vi "Write RFFE_w_Waveform.vi"(7 "Pins":string[](array[string])=["CLK", "SDA"], 8 "error in (no error)":errorcluster, 9 "Reg_Address_Data":T2={"Address"=81, "Data"=0} {"Address" format="%.0x"}, 10 "USID":T3 max=15, 11 "Semiconductor Module Context":T4) -> (0 "error out":errorcluster)   [LabVIEW 2013]
uses:
  <vilib>/NI_TestStand_SemiconductorModule/NI_TestStand_Semiconductor_Module.lvlibp/PinMap/General/SemiconductorModuleContext.ctl
  Controls/USID.ctl
  Controls/Reg_Address_Data.ctl
  MIPI_RFFE/Ctrls/RegReadWrite.ctl
  MIPI_RFFE/Ctrls/Configuration.ctl
  MIPI_RFFE/Ctrls/ClockDataChannels.ctl
  MIPI_RFFE/Ctrls/ExtendedRegReadWrite.ctl
  <instrlib>/niHSDIO/niHSDIO.llb/niHSDIO_ctl Generation Mode Values (Ring).ctl
  <vilib>/NI_TestStand_SemiconductorModule/NI_TestStand_Semiconductor_Module.lvlibp/PinMap/HSDIO/PinsToNIHSDIOSessions.vi
  <instrlib>/niHSDIO/niHSDIO.llb/niHSDIO Write Named Waveform (WDT).vi
  <vilib>/NI_TestStand_SemiconductorModule/NI_TestStand_Semiconductor_Module.lvlibp
panel:
  out "Converted Data":T1 {"Register" max=31 format="%.0x"; "Slave Address" max=15 format="%.0x"}
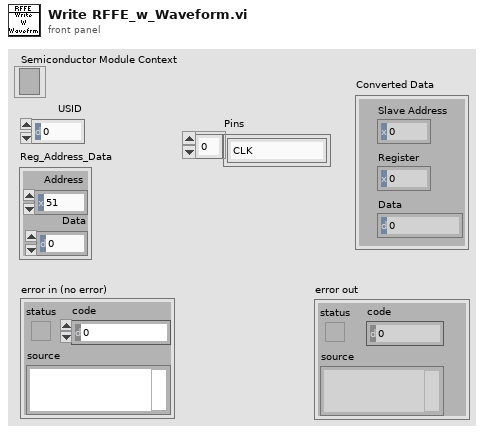
[diagram p1: front panel]
types:
  T1 = cluster{"Slave Address":u8, "Register":u8, "Data":u8}
  T2 = typedef "Reg_Address_Data.ctl" = cluster{"Address":u8, "Data":u8}
  T3 = typedef "USID.ctl" = u8
  T4 = typedef "NI_TestStand_Semiconductor_Module.lvlibp/SemiconductorModuleContext.ctl" = refnum<k7>
  T5 = typedef "Configuration.ctl" = cluster{"Samples to Allocate":i32, "Oversample Factor":u8, "Clock Channel":T6, "Data Channel":T6}
  T6 = typedef "ClockDataChannels.ctl" = enum16{"0", "1"}
  T7 = typedef "RegReadWrite.ctl" = cluster{"Slave Address":u8, "Register":u8, "Data":u8, "SetID_Pin_State":enum16{"0", "1", "Z"}}
  T8 = typedef "RFFE_Data.ctl" = cluster{"Clock Channel":T6, "Data Channel":T6, "Oversample Factor":u8, "Zero Array":u8[], "One Array":u8[], "Z Array ":u8[], "H Array":u8[], "L Array":u8[], "X Array":u8[], "Toggle (high to low)":u8[]}
  T9 = typedef "ExtendedRegReadWrite.ctl" = cluster{"Slave Address":u8, "Register":u8, "Data":u8[]}
  T10 = typedef "niHSDIO_ctl Generation Mode Values (Ring).ctl" = i32
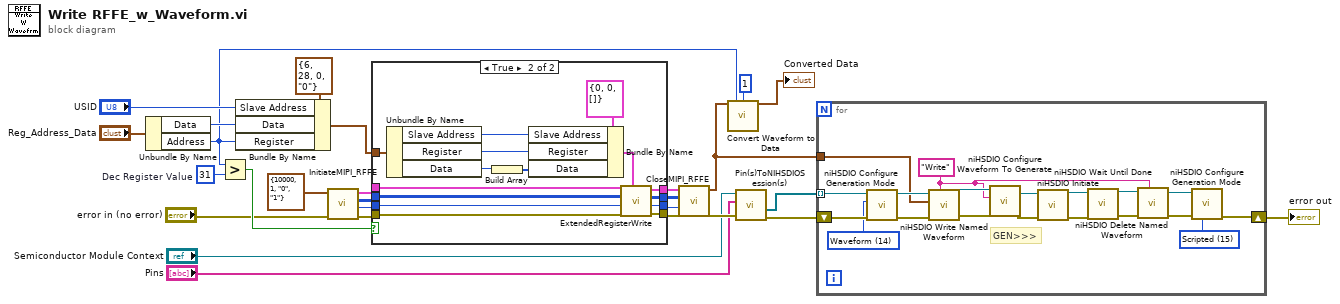
[diagram p0: block diagram]
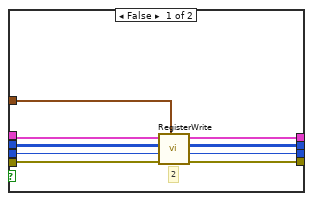
[diagram p2: hidden frame]
diagram:
  w23 = u8 31  # Dec Register Value
  n1 = Unbundle By Name("Reg_Address_Data") -> ("Data"=w5:u8, "Address"=w3:u8)
  n2 = Greater?(x=w3, y=w23) -> (0:w17:bool)
  n3 = Bundle By Name(cluster=T7 {"Slave Address"=6, "Register"=28, "Data"=0, "SetID_Pin_State"=enum."0"} ("Data"), "Slave Address"="USID", "Data"=w5, "Register"=w3) -> (w8:T7)
  n4 = call "InitiateMIPI_RFFE.vi"("error in (no error)"="error in (no error)", "Configuratation In"=T5 {"Samples to Allocate"=10000, "Oversample Factor"=1, "Clock Channel"=enum."0", "Data Channel"=enum."1"} ("Configuratation")) -> ("error out"=w16:errorcluster, "Number of Samples Out"=w15:i32, "Data Array"=w14:u8[][], "RFFE_Data"=w13:T8)  [unwired: 6 in]
  n5 = case shown="True" w17 {
    tunnel: [w31 w41] -> w22
    tunnel: [w30 w42] -> w21
    tunnel: [w29 w43] -> w20
    tunnel: [w28 w44] -> w19
    tunnel: w8 -> [w36 w50]
    tunnel: w16 -> [w32 w40]
    tunnel: w15 -> [w33 w39]
    tunnel: w14 -> [w34 w38]
    tunnel: w13 -> [w35 w37]
    frame False {
      # "2"
      n6 = call "RegisterWrite.vi"("Write Data"=w36, "error in (no error)"=w32, "Number of Samples In"=w33, "Data Array"=w34, "RFFE_Data"=w35) -> ("error out"=w28:errorcluster, "Number of Samples Out"=w29:i32, "Data Array Out"=w30:u8[][], "Configuratation Out"=w31:T8)  [unwired: 3 in]
    }
    frame True {
      n7 = Unbundle By Name(w50) -> ("Slave Address"=w49:u8, "Register"=w48:u8, "Data"=w47:u8)
      n8 = Build Array(w47) -> (w46:u8[])
      n9 = Bundle By Name(cluster=T9 {"Slave Address"=0, "Register"=0, "Data"=[]} ("Extended Read/Write"), "Slave Address"=w49, "Register"=w48, "Data"=w46) -> (w45:T9)
      n10 = call "ExtendedRegisterWrite.vi"("Extended Read/Write"=w45, "error in (no error)"=w40, "Number of Samples In"=w39, "Data Array"=w38, "RFFE_Data In"=w37) -> ("error out"=w44:errorcluster, "Number of Samples Out"=w43:i32, "Data Array Out"=w42:u8[][], "RFFE_Data Out"=w41:T8)  [unwired: 3 in]
    }
  }
  n11 = call "CloseMIPI_RFFE.vi"("error in (no error)"=w19, "Number of Samples"=w20, "Data Array"=w21, "RFFE_Data"=w22) -> ("error out"=w12:errorcluster, "Digital Waveform"=w4:digitalwaveform)  [unwired: 6 in]
  n12 = call "Convert Waveform to Data.vi"("Waveform Graph"=w4, "Register"=w3, "Ext_Read_Num_Reg"=u8 1) -> ("Converted Data"=→"Converted Data":T1)  [unwired: 10 in, 2 out]
  n13 = call-poly <vilib>:"Pin(s)ToNIHSDIOSession(s).vi"("error in (no error)"=w12, "Pins"="Pins", "Semiconductor Module Context"="Semiconductor Module Context") -> ("error out"=w26:errorcluster, "Generation Sessions"=w27:refnum<k15>[])  [unwired: 3 in, 4 out]
  n14 = for {
    tunnel: w27 -> [w68] mode=indexing
    shift-right: [w60] -> w24
    shift-left: w26 -> [w65]
    tunnel: w4 -> [w58]
    w59 = T10 15 items=["Waveform"=14, "Scripted"=15] ("generation mode (waveform)")
    w52 = "Write" ("waveform name (default:\"\")")
    w64 = T10 14 items=["Waveform"=14, "Scripted"=15] ("generation mode (waveform)")
    # "GEN>>>"
    n15 = call <instrlib>:"niHSDIO Configure Generation Mode.vi"("error in (no error)"=w65, "generation mode (waveform)"=w64, "instrument handle"=w68) -> ("error out"=w66:errorcluster, "instrument handle out"=w67:refnum<k15>)  [unwired: 7 in]
    n16 = call-poly <instrlib>:"niHSDIO Write Named Waveform.vi"("waveform name (default:\"\")"=w52, "error in (no error)"=w66, "data"=w58, "instrument handle"=w67) -> ("error out"=w63:errorcluster, "instrument handle out"=w62:refnum<k15>)  [unwired: 6 in]
    n17 = call <instrlib>:"niHSDIO Configure Waveform To Generate.vi"("error in (no error)"=w63, "waveform name"=w52, "instrument handle"=w62) -> ("error out"=w57:errorcluster, "instrument handle out"=w61:refnum<k15>)  [unwired: 7 in]
    n18 = call <instrlib>:"niHSDIO Initiate.vi"("error in (no error)"=w57, "instrument handle"=w61) -> ("error out"=w70:errorcluster, "instrument handle out"=w69:refnum<k15>)  [unwired: 8 in]
    n19 = call <instrlib>:"niHSDIO Wait Until Done.vi"("error in (no error)"=w70, "instrument handle"=w69) -> ("error out"=w56:errorcluster, "instrument handle out"=w53:refnum<k15>)  [unwired: 8 in]
    n20 = call <instrlib>:"niHSDIO Delete Named Waveform.vi"("waveform name (default:\"\")"=w52, "error in (no error)"=w56, "instrument handle"=w53) -> ("error out"=w55:errorcluster, "instrument handle out"=w54:refnum<k15>)  [unwired: 7 in]
    n21 = call <instrlib>:"niHSDIO Configure Generation Mode.vi"("error in (no error)"=w55, "generation mode (waveform)"=w59, "instrument handle"=w54) -> ("error out"=w60:errorcluster)  [unwired: 7 in, 1 out]
  }
  "error out" <- w24
